vi "Read Top caller.vi"(8 "error in (no error)":errorcluster, 11 "Mag Lab Measure Base in":refnum<class "Mag Lab Measure Base.lvclass">) -> (0 "error out":errorcluster, 2 "Top caller":bool, 3 "Mag Lab Measure Base out":refnum<class "Mag Lab Measure Base.lvclass">)   [LabVIEW 2015, in "Mag Lab Measure Base.lvclass"]
uses:
  Mag Lab Measure Base.lvclass
  Mag Lab Measure Base.lvclass/Mag Lab Measure Base.ctl
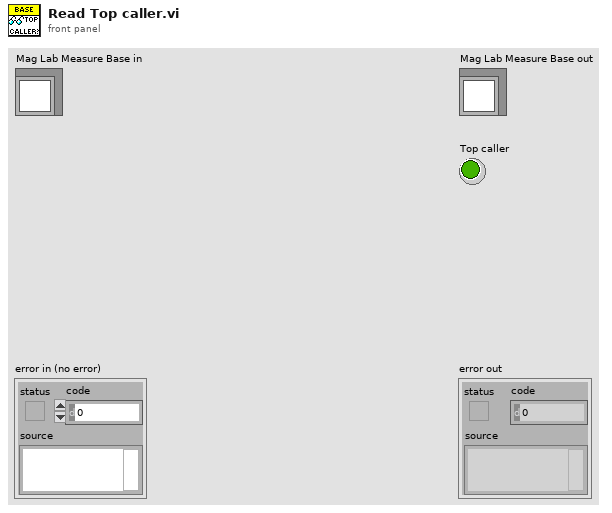
[diagram p1: front panel]
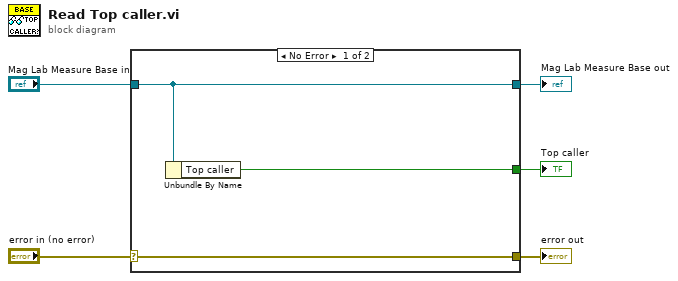
[diagram p0: block diagram]
diagram:
  n1 = case shown="No Error" "error in (no error)" {
    selector: "error in (no error)" -> [w8 w9]
    tunnel: [w8 w9] -> w4
    tunnel: [w7 w10] -> w2
    tunnel: "Mag Lab Measure Base in" -> [w7 w10]
    tunnel: [w6 _] -> w1
    frame No Error {
      n2 = Unbundle By Name(w7) -> ("Top caller"=w6:bool)
    }
    frame Error {
    }
  }
  "error out" <- w4
  "Mag Lab Measure Base out" <- w2
  "Top caller" <- w1
